vi "State.vi"(8 "error in":errorcluster, 10 "State":string) -> (0 "error out":errorcluster)   [LabVIEW 2019, in "Allmotion.lvlib"]
uses:
  Allmotion.lvlib
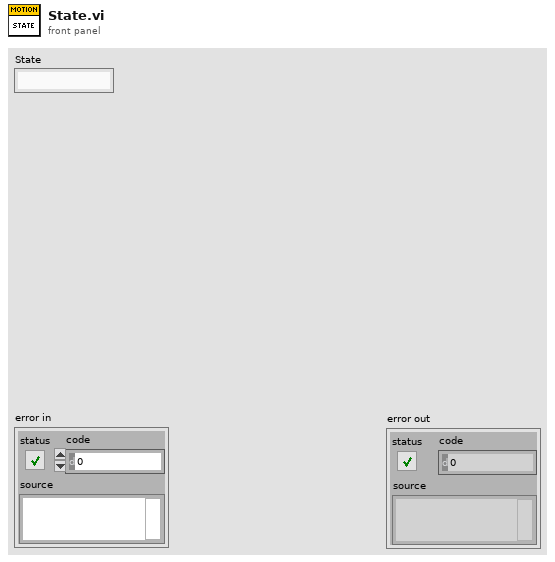
[diagram p1: front panel]
types:
  T1 = typedef "Allmotion.lvlib/SEQ Data.ctl" = cluster{"Position":i32[], "Arrived?":bool, "VISA name":refnum<visa-resource-name>, "Initialize Done?":bool, "State":string, "VI Refnum":refnum<vi>, "Dichroic Position":string[]}
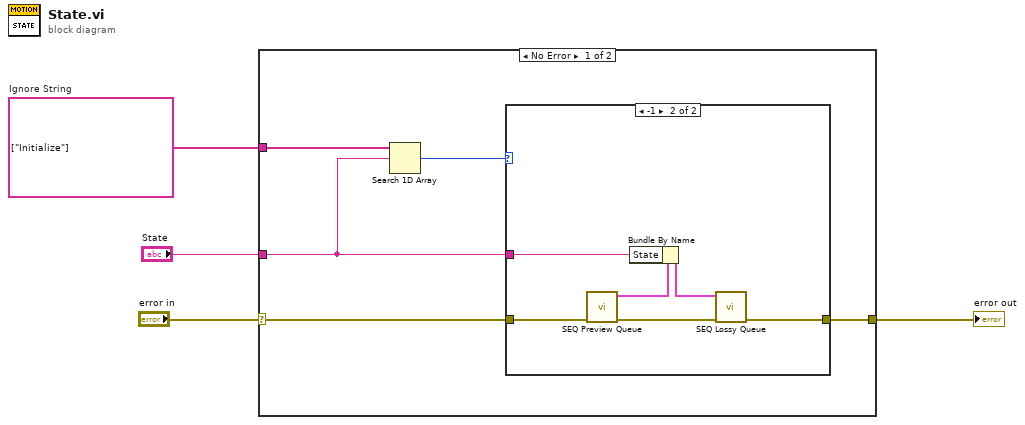
[diagram p0: block diagram]
diagram:
  w2 = string[] ["Initialize"]  # Ignore String
  n1 = case shown="No Error" "error in" {
    selector: "error in" -> [w9 w17]
    tunnel: [w8 w17] -> w3
    tunnel: w2 -> [w7 _]
    tunnel: "State" -> [w5 _]
    frame No Error {
      n2 = Search 1D Array(1D array=w7, element=w5) -> (index of element=w6:i32)  [unwired: 1 in]
      n3 = case shown="-1" w6 {
        tunnel: w9 -> [w10 w14]
        tunnel: [w10 w13] -> w8
        tunnel: w5 -> [_ w11]
        frame Default {
        }
        frame -1 {
          n4 = call "SEQ Preview Queue.vi"("error in"=w14) -> ("error out"=w16:errorcluster, "SEQ Data"=w15:T1)  [unwired: 9 in]
          n5 = Bundle By Name(cluster=w15, "State"=w11) -> (w12:T1)
          n6 = call "SEQ Lossy Queue.vi"("error in"=w16, "SEQ Data"=w12) -> ("error out"=w13:errorcluster)  [unwired: 9 in]
        }
      }
    }
    frame Error {
    }
  }
  "error out" <- w3
